vi "UDP Data Link - Configuration Utilities - Evaluate Rx Imported Channels.vi"(8 "error in (no error)":errorcluster, 9 "Section Info":T1, 10 "Channel Info Array":T2[](array[typedef]) {"Data Type" items=["U8", "U16", "U32", "U64", "I8", "I16", "I32", "I64", "SGL", "DBL", "EXT"]}, 11 "Node Ptr in":u64 format="%.0x") -> (0 "error out":errorcluster, 2 "Invalid Channels":string[](array[string]), 3 "Node Ptr out":u64 format="%.0x")   [LabVIEW 2015, in "UDP Data Link System Explorer.lvlib"]
uses:
  UDP Data Link System Explorer.lvlib
  TypeDefs/UDP Data Link - TypeDefs - XML Channel.ctl
  TypeDefs/UDP Data Link - TypeDefs - Section Info.ctl
  <vilib>/NI Veristand/Custom Device API/Custom Device Item Ref.ctl
  <vilib>/NI Veristand/Custom Device Tools/Custom Device Utility Library/NI VeriStand - Search for Item by GUID.vi
  <vilib>/NI Veristand/Custom Device API/Get Item Property (String Array).vi
  <vilib>/NI Veristand/Custom Device API/Set Item Property (String Array).vi
  <vilib>/NI Veristand/Custom Device Tools/Custom Device Utility Library/Custom Device Utility Library.lvlib
  <vilib>/NI Veristand/Custom Device API/Custom Device API.lvlib
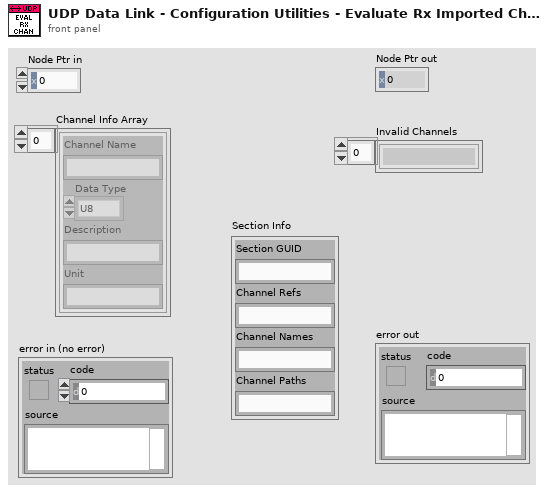
[diagram p1: front panel]
types:
  T1 = typedef "UDP Data Link System Explorer.lvlib/UDP Data Link - TypeDefs - Section Info.ctl" = cluster{"Section GUID":string, "Channel Refs":string, "Channel Names":string, "Channel Paths":string}
  T2 = typedef "UDP Data Link System Explorer.lvlib/UDP Data Link - TypeDefs - XML Channel.ctl" = cluster{"Channel Name":string, "Data Type":u16, "Description":string, "Unit":string}
  T3 = typedef "Custom Device API.lvlib/Custom Device Item Ref.ctl" = u64
  T4 = cluster{"Channel Names":string[], "Channel Paths":string[], "Dependent Node References":T3[]}
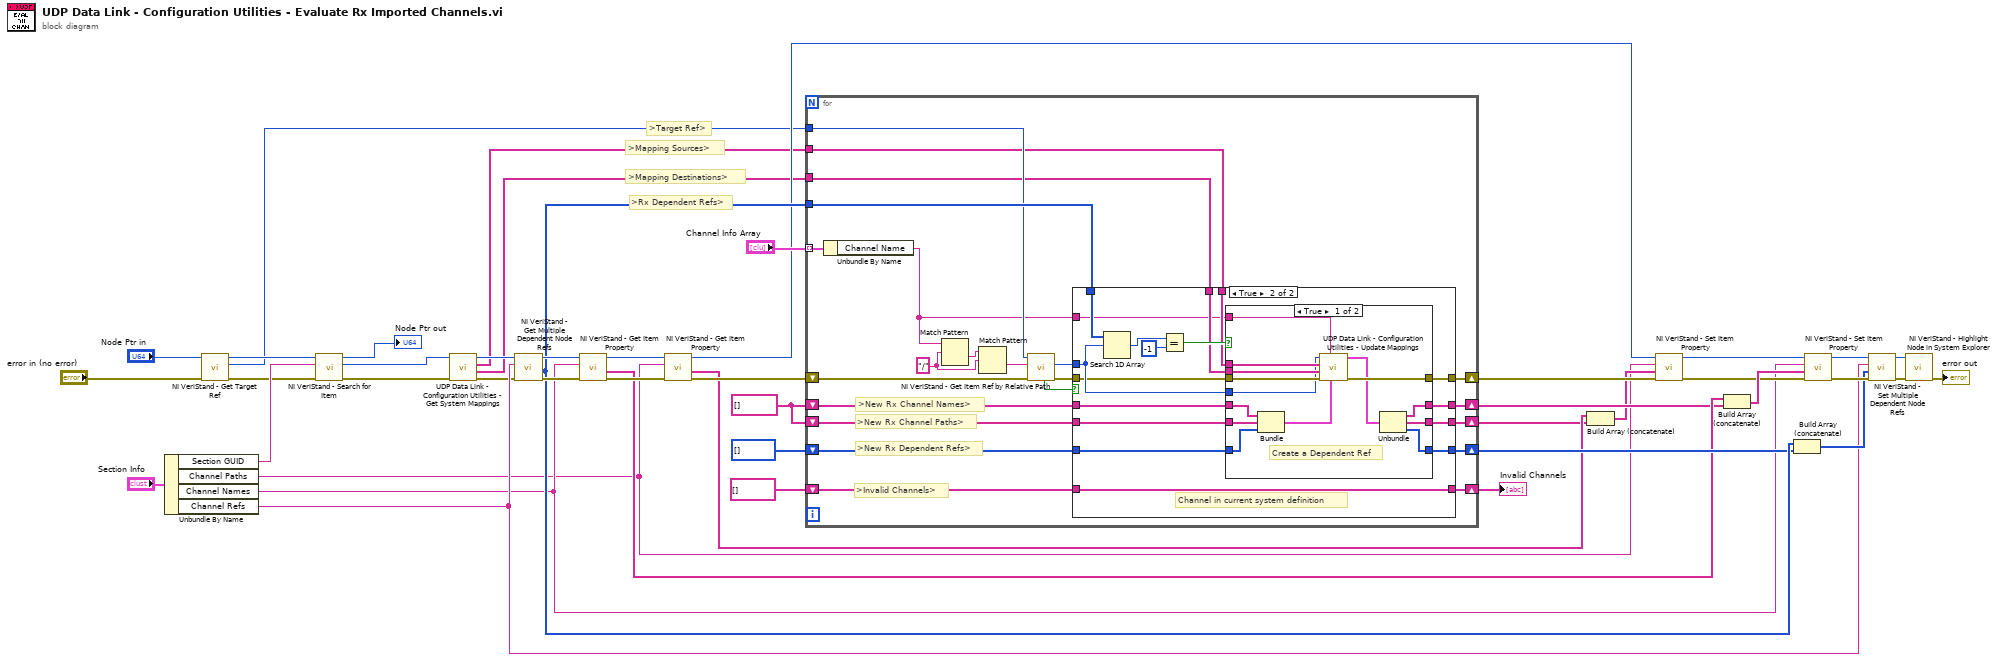
[diagram p0: block diagram]
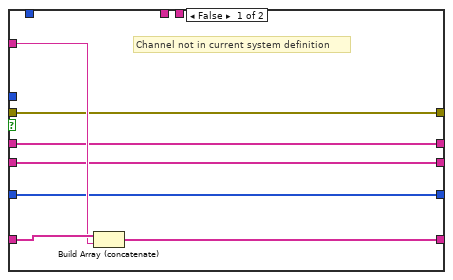
[diagram p2: hidden frame]
diagram:
  w35 = string[] []
  # ">Rx Dependent Refs>"
  # ">Mapping Destinations>"
  # ">Mapping Sources>"
  # ">Target Ref>"
  n1 = Unbundle By Name("Section Info") -> ("Section GUID"=w15:string, "Channel Paths"=w12:string, "Channel Names"=w13:string, "Channel Refs"=w14:string)
  n2 = call <vilib>:"NI VeriStand - Get Target Ref.vi"("error in"="error in (no error)", "Item Ref in"="Node Ptr in") -> ("error out"=w10:errorcluster, "Target Ref"=w7:T3, "Item Ref out"=w8:T3)  [unwired: 6 in, 1 out]
  n3 = call-poly <vilib>:"NI VeriStand - Search for Item.vi"("error in"=w10, "Item GUID"=w15, "Section Ref in"=w8) -> ("error out"=w5:errorcluster, "Item Ref"=w6:T3, "Section Ref out"=→"Node Ptr out":T3)  [unwired: 5 in, 1 out]
  n4 = call "UDP Data Link - Configuration Utilities - Get System Mappings.vi"("error in (no error)"=w5, "Item Ref in"=w6) -> ("error out"=w4:errorcluster, "Channel Path Destinations"=w2:string[], "Channel Path Sources"=w1:string[], "Item Ref out"=w3:T3)  [unwired: 6 in]
  n5 = call <vilib>:"NI VeriStand - Get Multiple Dependent Node Refs.vi"("error in (no error)"=w4, "Base Property Name"=w14, "Item Ref in"=w3) -> ("error out"=w41:errorcluster, "Dependent Node Refs"=w34:T3[], "Item Ref out"=w40:T3)  [unwired: 6 in]
  n6 = call-poly <vilib>:"NI VeriStand - Get Item Property.vi"("error in (no error)"=w41, "Property Name"=w13, "Item Ref in"=w40) -> ("error out"=w39:errorcluster, "Value"=w32:string[], "Item Ref out"=w38:T3)  [unwired: 5 in, 1 out]
  n7 = call-poly <vilib>:"NI VeriStand - Get Item Property.vi"("error in (no error)"=w39, "Property Name"=w12, "Item Ref in"=w38) -> ("error out"=w37:errorcluster, "Value"=w30:string[], "Item Ref out"=w27:T3)  [unwired: 5 in, 1 out]
  n8 = for {
    tunnel: "Channel Info Array" -> [w67] mode=indexing
    shift-right: [w66] -> w28
    shift-left: w37 -> [w56]
    shift-right: [w64] -> w43
    shift-left: string[] [] -> [w65]
    tunnel: w34 -> [w63]
    shift-right: [w61] -> w33
    shift-left: T3[] [] -> [w62]
    shift-right: [w59] -> w31
    shift-left: w35 -> [w60]
    shift-right: [w57] -> w29
    shift-left: w35 -> [w58]
    tunnel: w7 -> [w54]
    tunnel: w2 -> [w47]
    tunnel: w1 -> [w46]
    w49 = "/" ("regular expression")
    # ">Invalid Channels>"
    # ">New Rx Channel Names>"
    # ">New Rx Channel Paths>"
    # ">New Rx Dependent Refs>"
    n9 = Unbundle By Name(w67) -> ("Channel Name"=w51:string)
    n10 = Match Pattern(string=w51, regular expression=w49) -> (after substring=w50:string)  [unwired: 1 in, 3 out]
    n11 = Match Pattern(string=w50, regular expression=w49) -> (after substring=w48:string)  [unwired: 1 in, 3 out]
    n12 = call <vilib>:"NI VeriStand - Get Item Ref by Relative Path.vi"("error in"=w56, "Relative Item Path"=w48, "Section Ref in"=w54) -> ("error out"=w55:errorcluster, "Item Ref"=w53:T3, "Found"=w52:bool)  [unwired: 5 in, 1 out]
    n13 = case shown="True" w52 {
      tunnel: w55 -> [w71 w83]
      tunnel: [w71 w78] -> w66
      tunnel: w65 -> [w74 w91]
      tunnel: w51 -> [w73 w75]
      tunnel: [w72 w91] -> w64
      tunnel: w63 -> [_ w90]
      tunnel: w53 -> [_ w85]
      tunnel: w62 -> [w70 w86]
      tunnel: [w70 w84] -> w61
      tunnel: w60 -> [w69 w82]
      tunnel: [w69 w81] -> w59
      tunnel: w58 -> [w68 w80]
      tunnel: [w68 w79] -> w57
      tunnel: w47 -> [_ w77]
      tunnel: w46 -> [_ w76]
      frame False {
        # "Channel not in current system definition"
        n14 = Build Array (concatenate)(w74, w73) -> (w72:string[])
      }
      frame True {
        # "Channel in current system definition"
        n15 = Search 1D Array(1D array=w90, element=w85) -> (index of element=w89:i32)  [unwired: 1 in]
        n16 = Equal?(x=w89, y=-1) -> (x = y?=w87:bool)
        n17 = case shown="True" w87 {
          tunnel: w86 -> [w102 w108]
          tunnel: w85 -> [w92 _]
          tunnel: [w95 w108] -> w84
          tunnel: w83 -> [w105 w109]
          tunnel: w82 -> [w104 w107]
          tunnel: [w97 w107] -> w81
          tunnel: w80 -> [w103 w106]
          tunnel: [w96 w106] -> w79
          tunnel: [w99 w109] -> w78
          tunnel: w77 -> [w100 _]
          tunnel: w76 -> [w101 _]
          tunnel: w75 -> [w93 _]
          frame True {
            # "Create a Dependent Ref"
            n18 = Bundle(w104, w103, w102) -> (w94:cluster{string[], string[], T3[]})  [unwired: 1 in]
            n19 = call "UDP Data Link - Configuration Utilities - Update Mappings.vi"("Channel Data in"=w94, "Channel Path"=w93, "error in (no error)"=w105, "Channel Path Destinations"=w100, "Channel Path Sources"=w101, "Item Ref in"=w92) -> ("error out"=w99:errorcluster, "Channel Data out"=w98:T4)  [unwired: 4 in]
            n20 = Unbundle(w98) -> ("Channel Names"=w97:string[], "Channel Paths"=w96:string[], "Dependent Node References"=w95:T3[])
          }
          frame False {
            # "Channel is a Dependent Ref"
          }
        }
      }
    }
  }
  "Invalid Channels" <- w43
  n21 = Build Array (concatenate)(w30, w29) -> (w26:string[])
  n22 = call-poly <vilib>:"NI VeriStand - Set Item Property.vi"("error in (no error)"=w28, "Value"=w26, "Property Name"=w12, "Item Ref in"=w27) -> ("error out"=w23:errorcluster, "Item Ref out"=w25:T3)  [unwired: 5 in, 1 out]
  n23 = Build Array (concatenate)(w32, w31) -> (w24:string[])
  n24 = Build Array (concatenate)(w34, w33) -> (w20:T3[])
  n25 = call-poly <vilib>:"NI VeriStand - Set Item Property.vi"("error in (no error)"=w23, "Value"=w24, "Property Name"=w13, "Item Ref in"=w25) -> ("error out"=w22:errorcluster, "Item Ref out"=w21:T3)  [unwired: 5 in, 1 out]
  n26 = call <vilib>:"NI VeriStand - Set Multiple Dependent Node Refs.vi"("error in (no error)"=w22, "Dependent Node Refs"=w20, "Base Property Name"=w14, "Item Ref in"=w21) -> ("error out"=w19:errorcluster, "Item Ref out"=w18:T3)  [unwired: 6 in]
  n27 = call <vilib>:"NI VeriStand - Highlight Node in System Explorer.vi"("error in (no error)"=w19, "Item Ref in"=w18) -> ("error out"=→"error out":errorcluster)  [unwired: 8 in, 1 out]
